vi "Re-Broadcast Result.vi"(8 "error in (no error)":errorcluster, 10 "Acquired Result.lvclass":refnum<class "Acquired Result.lvclass">, 11 "Measure Controller in":refnum<class "Measure Controller.lvclass">) -> (0 "error out":errorcluster, 3 "Measure Controller out":refnum<class "Measure Controller.lvclass">)   [LabVIEW 2015, in "Measure Controller.lvclass"]
uses:
  Measure Controller.lvclass
  Results/Acquired Result/Acquired Result.lvclass
  Results/Acquired Result/Acquired Result.lvclass/Acquired Result.ctl
  Measure Object Messages/Broadcast Response Msg/Broadcast Response Msg.lvclass/Broadcast Response Msg.ctl
  <vilib>/ActorFramework/Message Enqueuer/Message Enqueuer.lvclass/Message Enqueuer.ctl
  Results/Acquired Result/Read Sender.vi
  <vilib>/ActorFramework/Message Enqueuer/Enqueue.vi
  <vilib>/ActorFramework/Message Priority Queue/Priority Enqueue.vi
  Measure Object Messages/Broadcast Response Msg/Broadcast Response Msg.lvclass
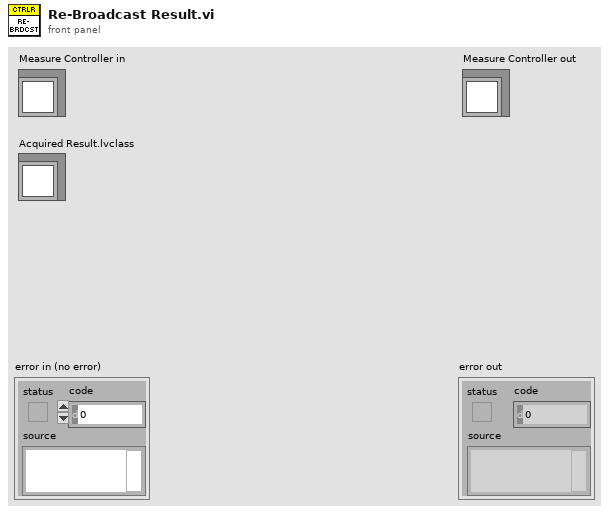
[diagram p1: front panel]
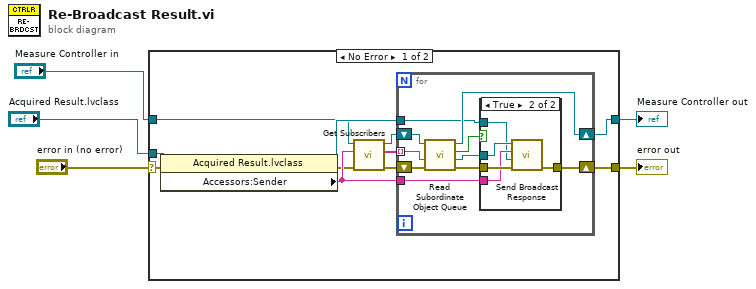
[diagram p0: block diagram]
diagram:
  n1 = case shown="No Error" "error in (no error)" {
    selector: "error in (no error)" -> [w9 w34]
    tunnel: [w8 w34] -> w4
    tunnel: [w6 w33] -> w2
    tunnel: "Measure Controller in" -> [w7 w33]
    tunnel: "Acquired Result.lvclass" -> [w10 _]
    frame No Error {
      n2 = property class="Acquired Result.lvclass"(reference=w10, error in=w9) -> (reference out=w16:refnum<class "Acquired Result.lvclass">, error out=w11:errorcluster, "Accessors:Sender"=w15:string)
      n3 = call-dynamic "Get Subscribers.vi"("error in (no error)"=w11, "Topic"=w15, "Measure Object in"=w7) -> ("error out"=w14:errorcluster, "Subscribers"=w13:string[], "Measure Object out"=w12:refnum<class "Measure Controller.lvclass">)  [unwired: 6 in]
      n4 = for {
        shift-right: [w23] -> w6
        shift-left: w12 -> [w26]
        tunnel: w13 -> [w25] mode=indexing
        shift-right: [w19] -> w8
        shift-left: w14 -> [w24]
        tunnel: w15 -> [w18]
        tunnel: w16 -> [w17]
        n5 = call-dynamic "Read Subordinate Object Queue.vi"("error in (no error)"=w24, "Name"=w25, "Measure Object in"=w26) -> ("error out"=w20:errorcluster, "Object Enqueuer"=w22:refnum<class "Message Enqueuer.lvclass">, "Found?"=w21:bool, "Measure Object out"=w23:refnum<class "Measure Controller.lvclass">)  [unwired: 5 in]
        n6 = case shown="True" w21 {
          tunnel: w22 -> [_ w32]
          tunnel: w20 -> [w27 w31]
          tunnel: [w27 w30] -> w19
          tunnel: w18 -> [_ w29]
          tunnel: w17 -> [_ w28]
          frame False {
          }
          frame True {
            n7 = call "Send Broadcast Response.vi"("error in (no error)"=w31, "Acquired Result.lvclass"=w28, "Topic"=w29, "Message Enqueuer"=w32) -> ("error out"=w30:errorcluster)  [unwired: 6 in, 1 out]
          }
        }
      }
    }
    frame Error {
    }
  }
  "error out" <- w4
  "Measure Controller out" <- w2
